vi "Start.vi"(8 "error in (no error)":errorcluster, 11 "Sample Study PID in":refnum<class "Sample Study PID.lvclass">) -> (0 "error out":errorcluster, 3 "Sample Study PID out":refnum<class "Sample Study PID.lvclass">)   [LabVIEW 2023, in "Sample Study PID.lvclass"]
uses:
  Sample Study PID.lvclass
  Sample Study PID.lvclass/Sample Study PID.ctl
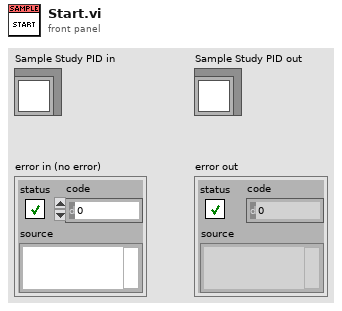
[diagram p1: front panel]
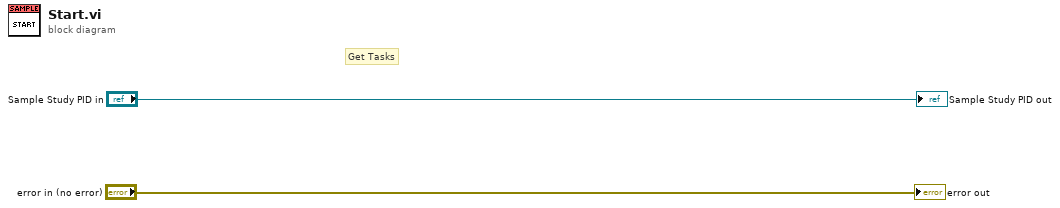
[diagram p0: block diagram]
diagram:
  # "Get Tasks"
  "error out" <- "error in (no error)"
  "Sample Study PID out" <- "Sample Study PID in"
